vi "Close Excel Ref.vi"(8 "error in":errorcluster, 11 "excelRefs in":T1) -> (0 "error out":errorcluster)   [LabVIEW 2020]
uses:
  Controls/excelRefContainer.ctl
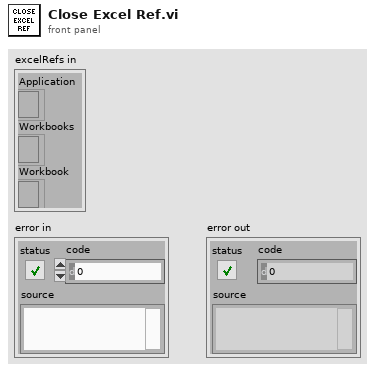
[diagram p1: front panel]
types:
  T1 = typedef "excelRefContainer.ctl" = cluster{"Application":refnum<k7>, "Workbooks":refnum<k7>, "Workbook":refnum<k7>}
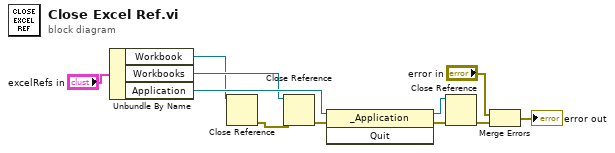
[diagram p0: block diagram]
diagram:
  n1 = Unbundle By Name("excelRefs in") -> ("Workbook"=w2:refnum<k7>, "Workbooks"=w6:refnum<k7>, "Application"=w7:refnum<k7>)
  n2 = Close Reference(reference=w2) -> (error out=w1:errorcluster)  [unwired: 1 in]
  n3 = Close Reference(reference=w6, error in (no error)=w1) -> (error out=w10:errorcluster)
  n4 = invoke class="_Application" method="Quit"(reference=w7, error in=w10) -> (reference out=w11:refnum<k7>, error out=w9:errorcluster)  [unwired: 1 in, 1 out]
  n5 = Close Reference(reference=w11, error in (no error)=w9) -> (error out=w4:errorcluster)
  n6 = Merge Errors("error in", w4) -> (→"error out":errorcluster)
